vi "SRX_Send Point.vi"(7 "Point Array":T6[](array[typedef]), 8 "Error":errorcluster, 10 "Index":i32, 11 "CAN Talon SRX Ref":T1={"DeviceStatus"={"status"=FALSE, "code"=0, "source"=""}, "Type"=enum."PWM", "PWM"={"PWM Channel"=enum."PWM 0", "DeadBand"={"Name"="", "maxPositivePwm"=0, "minPositivePwm"=0, "centerPwm"=0, "maxNegativePwm"=0, "minNegativePwm"=0, "angularRange"=0}}, "CAN"={"Device Number"=0, "SetOutput VI Ref"=variant, "GetOutput VI Ref"=variant, "Enable VI Ref"=variant, "Disable VI Ref"=variant, "Data"=variant}, "Invert"=FALSE, "DIO PWM"={"PWM \"Enable\" Channel"=enum."Invalid", "DIOChannel"=enum."Invalid", "PWM Rate"=0.0}}) -> (0 "Error Out":errorcluster, 1 "Last Point Out":bool, 2 "Next Index Out":i32, 3 "CAN Talon SRX Ref Out":T1={"DeviceStatus"={"status"=FALSE, "code"=0, "source"=""}, "Type"=enum."PWM", "PWM"={"PWM Channel"=enum."PWM 0", "DeadBand"={"Name"="", "maxPositivePwm"=0, "minPositivePwm"=0, "centerPwm"=0, "maxNegativePwm"=0, "minNegativePwm"=0, "angularRange"=0}}, "CAN"={"Device Number"=0, "SetOutput VI Ref"=variant, "GetOutput VI Ref"=variant, "Enable VI Ref"=variant, "Disable VI Ref"=variant, "Data"=variant}, "Invert"=FALSE, "DIO PWM"={"PWM \"Enable\" Channel"=enum."Invalid", "DIOChannel"=enum."Invalid", "PWM Rate"=0.0}}, 5 "Buffer Full Out":bool)   [LabVIEW 2017]
uses:
  TypeDef/CLUSTER_Drive_Point Specification.ctl
  <vilib>/Rock Robotics/WPI/MotorControl/WPI_MotorControlDeviceRef.ctl
  <vilib>/Rock Robotics/WPI/MotorControl/WPI_MotorControlType.ctl
  <vilib>/Rock Robotics/SystemInterfaces/DIO/FPGA_DIOPWMChannel.ctl
  <vilib>/Rock Robotics/WPI/PWM/WPI_PWMDeadband.ctl
  <vilib>/Rock Robotics/SystemInterfaces/DIO/FPGA_DIOChannel.ctl
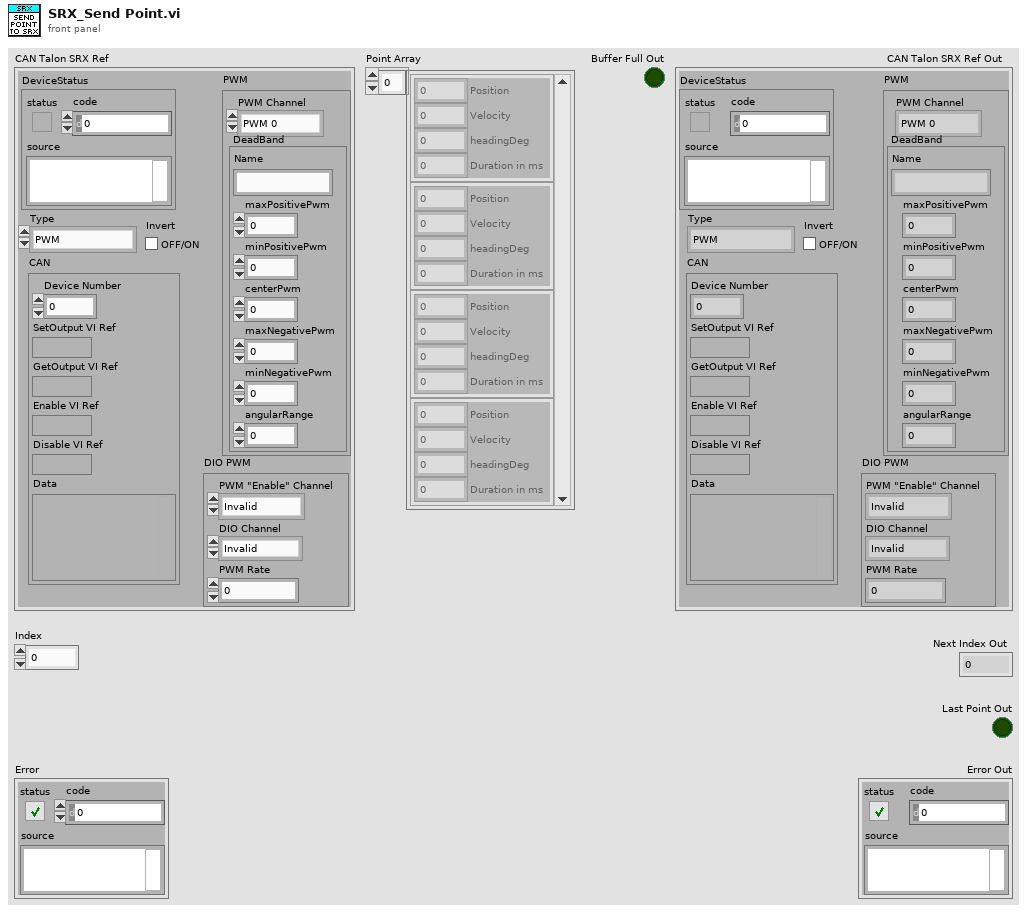
[diagram p1: front panel]
types:
  T1 = typedef "WPI_MotorControlDeviceRef.ctl" = cluster{"DeviceStatus":errorcluster, "Type":T2, "PWM":cluster{"PWM Channel":T3, "DeadBand":T4}, "CAN":cluster{"Device Number":u8, "SetOutput VI Ref":variant, "GetOutput VI Ref":variant, "Enable VI Ref":variant, "Disable VI Ref":variant, "Data":variant}, "Invert":bool, "DIO PWM":cluster{"PWM \"Enable\" Channel":T3, "DIOChannel":T5, "PWM Rate":dbl}}
  T2 = typedef "WPI_MotorControlType.ctl" = enum16{"PWM", "CAN", "DIO PWM"}
  T3 = typedef "FPGA_DIOPWMChannel.ctl" = enum8{"PWM 0", "PWM 1", "PWM 2", "PWM 3", "PWM 4", "PWM 5", "PWM 6", "PWM 7", "PWM 8", "PWM 9", "PWM MXP 0", "PWM MXP 1", "PWM MXP 2", "PWM MXP 3", "PWM MXP 4", "PWM MXP 5", "PWM MXP 6", "PWM MXP 7", "PWM MXP 8", "PWM MXP 9", "Invalid"}
  T4 = typedef "WPI_PWMDeadband.ctl" = cluster{"Name":string, "maxPositivePwm":i32, "minPositivePwm":i32, "centerPwm":i32, "maxNegativePwm":i32, "minNegativePwm":i32, "angularRange":u16}
  T5 = typedef "FPGA_DIOChannel.ctl" = enum8{"DIO 0", "DIO 1", "DIO 2", "DIO 3", "DIO 4", "DIO 5", "DIO 6", "DIO 7", "DIO 8", "DIO 9", "DIO MXP 0", "DIO MXP 1", "DIO MXP 2", "DIO MXP 3", "DIO MXP 4", "DIO MXP 5", "DIO MXP 6", "DIO MXP 7", "DIO MXP 8", "DIO MXP 9", "DIO MXP 10", "DIO MXP 11", "DIO MXP 12", "DIO MXP 13", "DIO MXP 14", "DIO MXP 15", "SPI Port CS1", "SPI Port CS2", "SPI Port CS3", "SPI Port MISO", "SPI Port MOSI", "Invalid"}
  T6 = typedef "CLUSTER_Drive_Point Specification.ctl" = cluster{"Position":dbl, "Velocity":dbl, "headingDeg":dbl, "Duration in ms":i32}
  T7 = cluster{"Top Buffer Remaining":i32, "Top Buffer Count":i32, "Bottom Buffer Count":i32, "Has Underrun?":bool, "Is Underrun?":bool, "Active Point Valid?":bool, "Is Last?":bool, "Profile Slot Select 0":i32, "Output Enable":i32, "Time Duration (ms)":i32, "Profile Slot Select 1":i32}
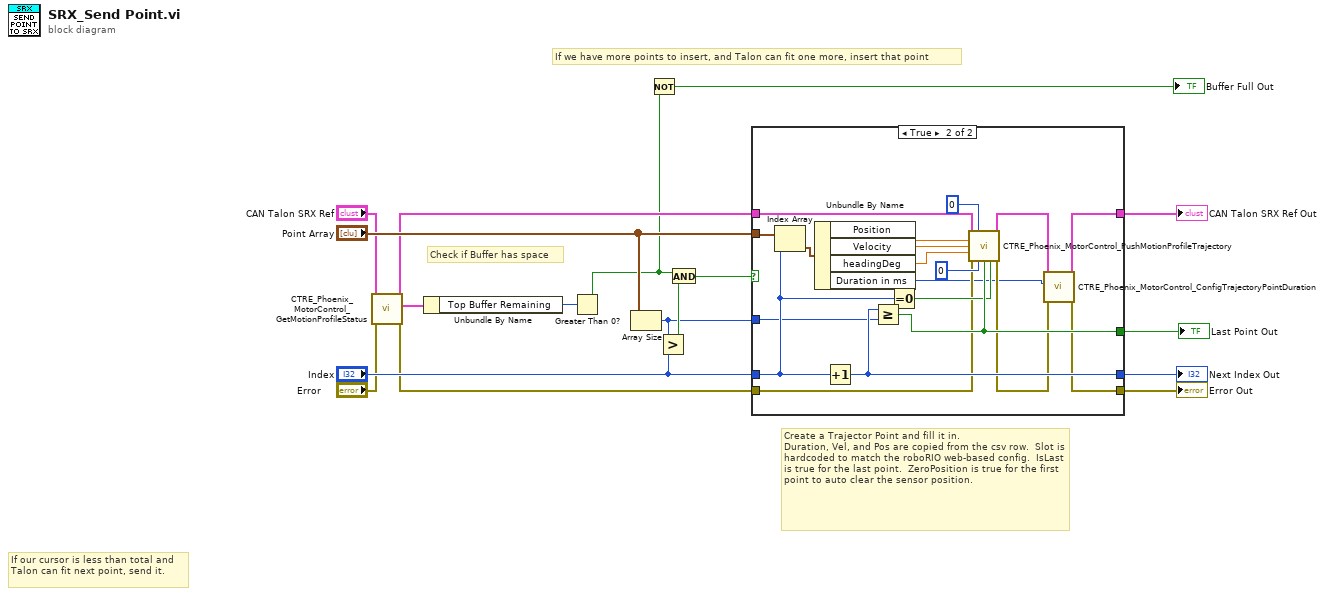
[diagram p0: block diagram]
diagram:
  # "Check if Buffer has space"
  # "Create a Trajector Point and fill it in.\nDuration, Vel, and Pos are copied from the csv row.  Slot is hardcoded to match the roboRIO web-based config.  IsLast is true for the last point.  ZeroPosition is true for the first point to auto clear the sensor position."
  # "If our cursor is less than total and Talon can fit next point, send it."
  # "If we have more points to insert, and Talon can fit one more, insert that point"
  n1 = call "CTRE_Phoenix_MotorControl_GetMotionProfileStatus.vi"("error in"="Error", "PhoenixMotorControlDevRef"="CAN Talon SRX Ref") -> ("error out"=w5:errorcluster, "Motion Profile Status"=w3:T7, "PhoenixMotorControlDevRef"=w6:T1)  [unwired: 7 in]
  n2 = Unbundle By Name(w3) -> ("Top Buffer Remaining"=w2:i32)
  n3 = Greater Than 0?(x=w2) -> (x > 0?=w1:bool)
  n4 = Array Size(array="Point Array") -> (size(s)=w9:i32)
  n5 = Not(x=w1) -> (.not. x?=→"Buffer Full Out":bool)
  n6 = Greater?(x=w9, y="Index") -> (0:w17:bool)
  n7 = And(x=w1, y=w17) -> (x .and. y?=w15:bool)
  n8 = case shown="True" w15 {
    tunnel: "Point Array" -> [_ w39]
    tunnel: [w20 w37] -> w14
    tunnel: "Index" -> [w20 w38]
    tunnel: w9 -> [_ w36]
    tunnel: w6 -> [w18 w34]
    tunnel: w5 -> [w19 w28]
    tunnel: [w19 w25] -> w13
    tunnel: [_ w30] -> w12
    tunnel: [w18 w22] -> w11
    frame False {
    }
    frame True {
      n9 = Index Array(array=w39, index=w38) -> (element=w35:T6)
      n10 = Unbundle By Name(w35) -> ("Position"=w33:dbl, "Velocity"=w32:dbl, "headingDeg"=w27:dbl, "Duration in ms"=w24:i32)
      n11 = Increment(x=w38) -> (x+1=w37:i32)
      n12 = Greater Or Equal?(x=w37, y=w36) -> (x >= y?=w30:bool)
      n13 = Equal To 0?(x=w38) -> (x = 0?=w29:bool)
      n14 = call "CTRE_Phoenix_MotorControl_PushMotionProfileTrajectory.vi"("PhoenixMotorControlDevRef"=w34, "profileSlotSelect1"=0, "position"=w33, "velocity"=w32, "headingDeg"=w27, "error in"=w28, "profileSlotSelect0"=0 ("profileSlotSelect"), "isLastPoint?"=w30, "Zero Position?"=w29) -> ("PhoenixMotorControlDevRef"=w23:T1, "error out"=w26:errorcluster)  [unwired: 5 in]
      n15 = call "CTRE_Phoenix_MotorControl_ConfigTrajectoryPointDuration.vi"("error in"=w26, "durationMs"=w24, "PhoenixMotorControlDevRef"=w23) -> ("error out"=w25:errorcluster, "PhoenixMotorControlDevRef"=w22:T1)  [unwired: 7 in]
    }
  }
  "Next Index Out" <- w14
  "CAN Talon SRX Ref Out" <- w11
  "Error Out" <- w13
  "Last Point Out" <- w12
